vi "Begin.vi"(8 "error in (no error)":errorcluster, 11 "Compressor in":refnum<class "Compressor.lvclass">) -> (0 "error out":errorcluster, 3 "Compressor out":refnum<class "Compressor.lvclass">)   [LabVIEW 2013, in "Compressor.lvclass"]
uses:
  Compressor.lvclass
  <vilib>/Rock Robotics/SystemInterfaces/Typedef/FPGA_TypedefDigitalModule.ctl
  <vilib>/Rock Robotics/SystemInterfaces/DIO/FPGA_DIOChannel.ctl
  <vilib>/Rock Robotics/SystemInterfaces/DIO/FPGA_DIORelayChannel.ctl
  System/System.lvclass
panel:
  in  "Relay Channel":T1=enum."Relay 2"
  in  "Relay Digital Module (Module 1)":T2
  in  "Pressure Switch DIO Channel":T3=enum."DIO 3"
  in  "Pressure Switch Digital Module (Module 1)":T2
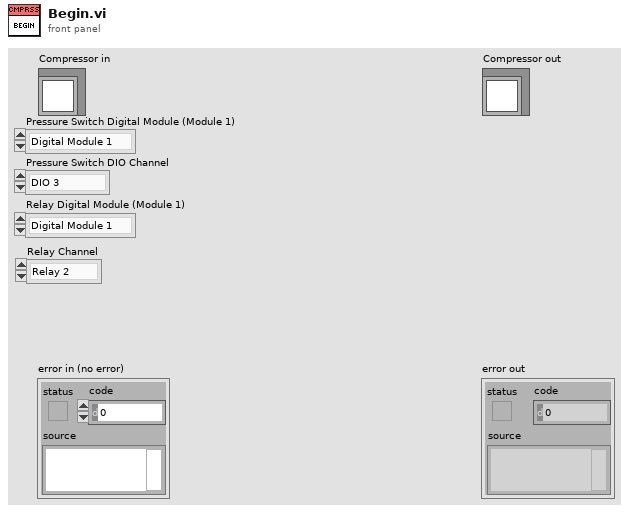
[diagram p1: front panel]
types:
  T1 = typedef "FPGA_DIORelayChannel.ctl" = enum8{"Relay 1", "Relay 2", "Relay 3", "Relay 4", "Relay 5", "Relay 6", "Relay 7", "Relay 8", "Invalid"}
  T2 = typedef "FPGA_TypedefDigitalModule.ctl" = enum16{"Digital Module 1", "Digital Module 2"}
  T3 = typedef "FPGA_DIOChannel.ctl" = enum8{"DIO 1", "DIO 2", "DIO 3", "DIO 4", "DIO 5", "DIO 6", "DIO 7", "DIO 8", "DIO 9", "DIO 10", "DIO 11", "DIO 12", "DIO 13", "DIO 14", "Invalid"}
  T4 = typedef "WPI_CompressorDevRef.ctl" = cluster{"DevStatus":errorcluster, "DigitalInputDevRef":T5, "RelayDevRef":T6}
  T5 = typedef "WPI_DigitalInputDevRef.ctl" = cluster{"DevStatus":errorcluster, "DIO Channel":T3, "Digital Module":T2}
  T6 = typedef "WPI_RelayDevRef.ctl" = cluster{"DevStatus":errorcluster, "Relay Channel":T1, "Digital Module":T2, "Relay Direction":T7}
  T7 = typedef "WPI_RelayDirection.ctl" = enum16{"Both directions", "Forward only", "Reverse only"}
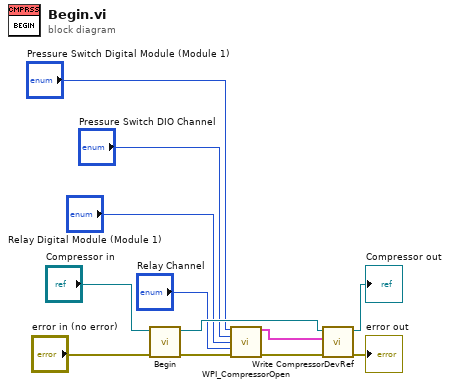
[diagram p0: block diagram]
diagram:
  n1 = call-parent "Begin.vi"("error in (no error)"="error in (no error)", "System in"="Compressor in") -> ("error out"=w4:errorcluster, "System out"=w9:refnum<class "Compressor.lvclass">)  [unwired: 8 in]
  n2 = call <vilib>:"WPI_CompressorOpen.vi"("Pressure Switch Digital Module (Module 1)"="Pressure Switch Digital Module (Module 1)", "Pressure Switch DIO Channel"="Pressure Switch DIO Channel", "Relay Digital Module (Module 1)"="Relay Digital Module (Module 1)", "Relay Channel"="Relay Channel", "error in (no error)"=w4) -> ("CompressorDevRef"=w2:T4, "error out"=w1:errorcluster)  [unwired: 9 in]
  n3 = call-dynamic "Write CompressorDevRef.vi"("error in (no error)"=w1, "CompressorDevRef"=w2, "Compressor in"=w9) -> ("error out"=→"error out":errorcluster, "Compressor out"=→"Compressor out":refnum<class "Compressor.lvclass">)  [unwired: 7 in]
